vi "Configure Trace (Reflection Measurement).vi"(7 "Enable Trace Average (T: Enable)":bool=TRUE, 8 "error in (no error)":errorcluster, 9 "Trace Average Number (1)":i32=1, 10 "Trace Math Type (4: None)":i32(ring)=4 items=["Off", "Data + Memory", "Data - Memory", "Data / Memory", "None"], 11 "VISA resource name":refnum<visa-resource-name>) -> (0 "error out":errorcluster, 3 "VISA resource name out":refnum<visa-resource-name>)   [LabVIEW 2022 SP3, in "Agilent N934X Series.lvlib"]
doc: "Configures the Trace settings of reflection measurement mode.\n\nNote:\nThis VI is only applicable for N9321C, N9322C, N9323C, N9324C models."
uses:
  <instrlib>/Agilent N934X Series/Agilent N934X Series.lvlib
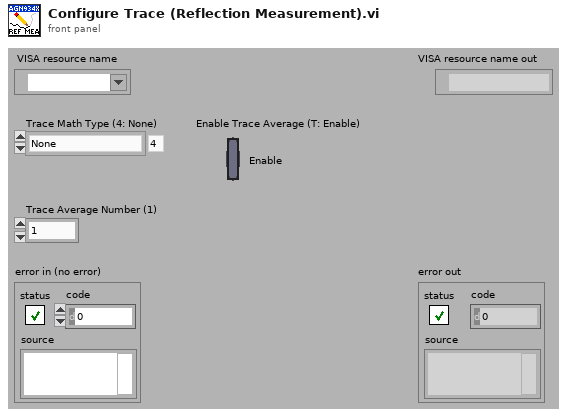
[diagram p1: front panel]
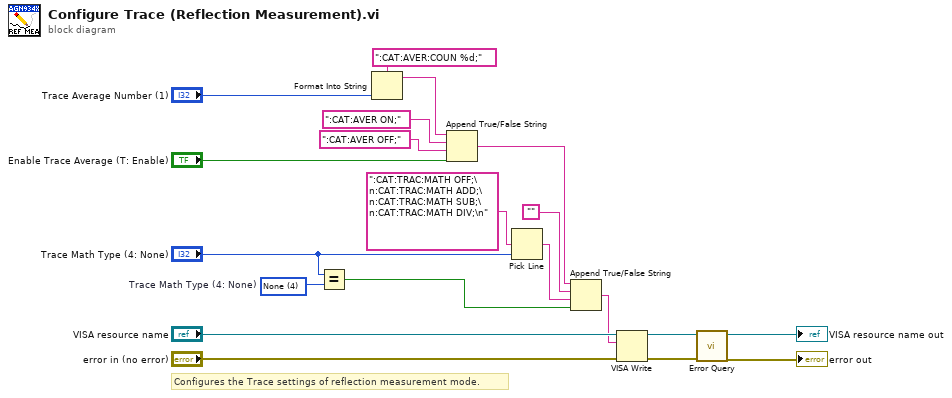
[diagram p0: block diagram]
diagram:
  w7 = 4 items=["Off", "Data + Memory", "Data - Memory", "Data / Memory", "None"]  # Trace Math Type (4: None)
  # "Configures the Trace settings of reflection measurement mode."
  n1 = Equal?(x="Trace Math Type (4: None)", y=w7) -> (x = y?=w4:bool)
  n2 = Format Into String(format string=":CAT:AVER:COUN %d;", "Trace Average Number (1)") -> (resulting string=w18:string)  [unwired: 2 in, 1 out]
  n3 = Append True/False String(1:"Enable Trace Average (T: Enable)", 2:":CAT:AVER OFF;", 3:":CAT:AVER ON;", 4:w18) -> (0:w3:string)
  n4 = Pick Line(multi-line string=":CAT:TRAC:MATH OFF;\n:CAT:TRAC:MATH ADD;\n:CAT:TRAC:MATH SUB;\n:CAT:TRAC:MATH DIV;\n", line index="Trace Math Type (4: None)") -> (output string=w2:string)  [unwired: 1 in]
  n5 = Append True/False String(1:w4, 2:w2, 3:"", 4:w3) -> (0:w5:string)
  n6 = VISA Write(VISA resource name="VISA resource name", write buffer=w5, error in (no error)="error in (no error)") -> (VISA resource name out=w11:refnum<visa-resource-name>, error out=w10:errorcluster)  [unwired: 1 out]
  n7 = call <instrlib>:"Error Query.vi"("error in (no error)"=w10, "VISA resource name"=w11) -> ("error out"=→"error out":errorcluster, "VISA resource name out"=→"VISA resource name out":refnum<visa-resource-name>)  [unwired: 6 in, 2 out]
